vi "Filter Drawings.vi"() -> ()   [LabVIEW 2025]
uses:
  <vilib>/Analysis/4window.llb/Gaussian Window (DBL).vi
  <vilib>/Analysis/NI_AALBase.lvlib
  <vilib>/Analysis/NI_AALPro.lvlib
panel:
  in  "n":i32
  in  "delay":dbl format="%#_13g"
  out "Waveform Graph":dbl[](graph)
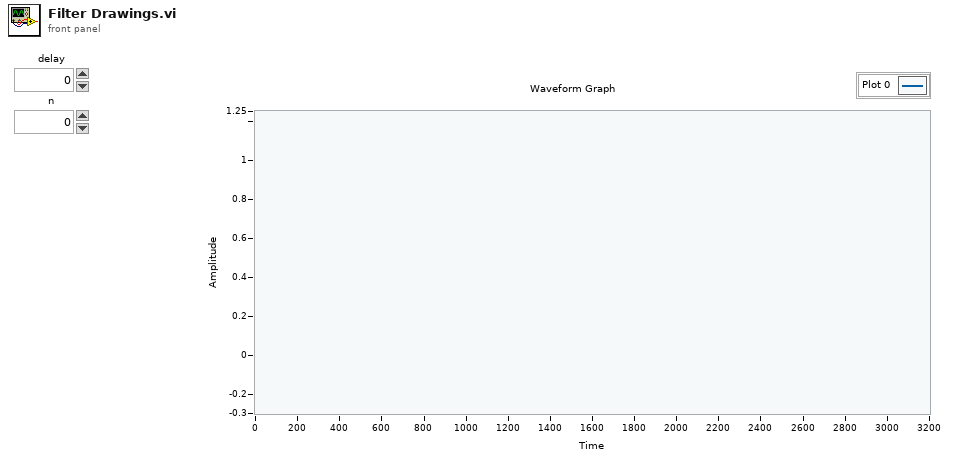
[diagram p1: front panel]
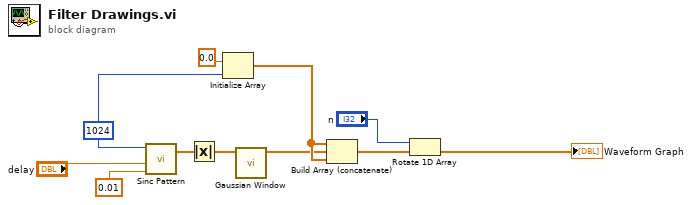
[diagram p0: block diagram]
diagram:
  w5 = 1024 ("samples")
  n1 = call <vilib>:"Sinc Pattern.vi"("delta t"=0.01, "delay"="delay", "samples"=w5) -> ("Sinc Pattern"=w11:dbl[])  [unwired: 1 in, 1 out]
  n2 = Absolute Value(x=w11) -> (abs(x)=w8:dbl[])
  n3 = Initialize Array(0.0 ("delta t"), w5) -> (w3:dbl[])
  n4 = call-poly <vilib>:"Gaussian Window.vi"("X"=w8) -> ("Windowed X"=w2:dbl[])  [unwired: 9 in, 1 out]
  n5 = Build Array (concatenate)(w3, w2, w3) -> (w1:dbl[])
  n6 = Rotate 1D Array(1:w1, 2:"n") -> (0:→"Waveform Graph":dbl[])
